vi "Periodic Tasks.vi"(8 "error in":errorcluster) -> (0 "error out":errorcluster)   [LabVIEW 2018]
doc: "This VI runs in parallel to other tasks. It can contain as many user-defined periodic loops as you need. These can carry out PID or other sorts of timed response."
uses:
  <vilib>/Rock Robotics/WPI/Joystick/WPI_JoystickDevRef.ctl
  <vilib>/Rock Robotics/WPI/Joystick/WPI_JoystickDeviceEnum.ctl
  <vilib>/Rock Robotics/WPI/RobotDrive/WPI_RobotDriveDevRef.ctl
  <vilib>/Rock Robotics/WPI/MotorControl/WPI_MotorControlDeviceRef.ctl
  <vilib>/Rock Robotics/WPI/MotorControl/WPI_MotorControlType.ctl
  <vilib>/Rock Robotics/SystemInterfaces/DIO/FPGA_DIOPWMChannel.ctl
  <vilib>/Rock Robotics/WPI/PWM/WPI_PWMDeadband.ctl
  <vilib>/Rock Robotics/SystemInterfaces/DIO/FPGA_DIOChannel.ctl
  <vilib>/Rock Robotics/WPI/Solenoid/WPI_SolenoidDevRef.ctl
  <vilib>/Rock Robotics/WPI/Solenoid/WPI_SolenoidChannel.ctl
  <vilib>/Rock Robotics/WPI/DriverStation/WPI_DriverStationRobotMode2.ctl
  Vision States.ctl
  <vilib>/Rock Robotics/WPI/Utilities/WPI_GetSetVariantRefNum.vi
  Robot Global Data.vi
  <vilib>/Rock Robotics/Network Tables/NT Write Number.vi
  <vilib>/Rock Robotics/Network Tables/NT Read Number.vi
panel:
  in  "RetainerSolenoidDevRef":T1={"DevStatus"={"status"=FALSE, "code"=0, "source"=""}, "Pneumatics Control Module"=0, "Forward Solenoid Channel"=enum."Invalid", "Reverse Solenoid Channel"=enum."Invalid"}
  in  "KickerSolenoidDevRef":T1={"DevStatus"={"status"=FALSE, "code"=0, "source"=""}, "Pneumatics Control Module"=0, "Forward Solenoid Channel"=enum."Invalid", "Reverse Solenoid Channel"=enum."Invalid"}
  in  "Drive Motors":T3={"DevStatus"={"status"=FALSE, "code"=0, "source"=""}, "Motors[]"=[], "Square Inputs"=FALSE, "Max Output"=1.0}
  in  "AuxJoystickDevRef":T9={"Device"=enum."USB 1"}
  in  "DriveJoystickDevRef":T9
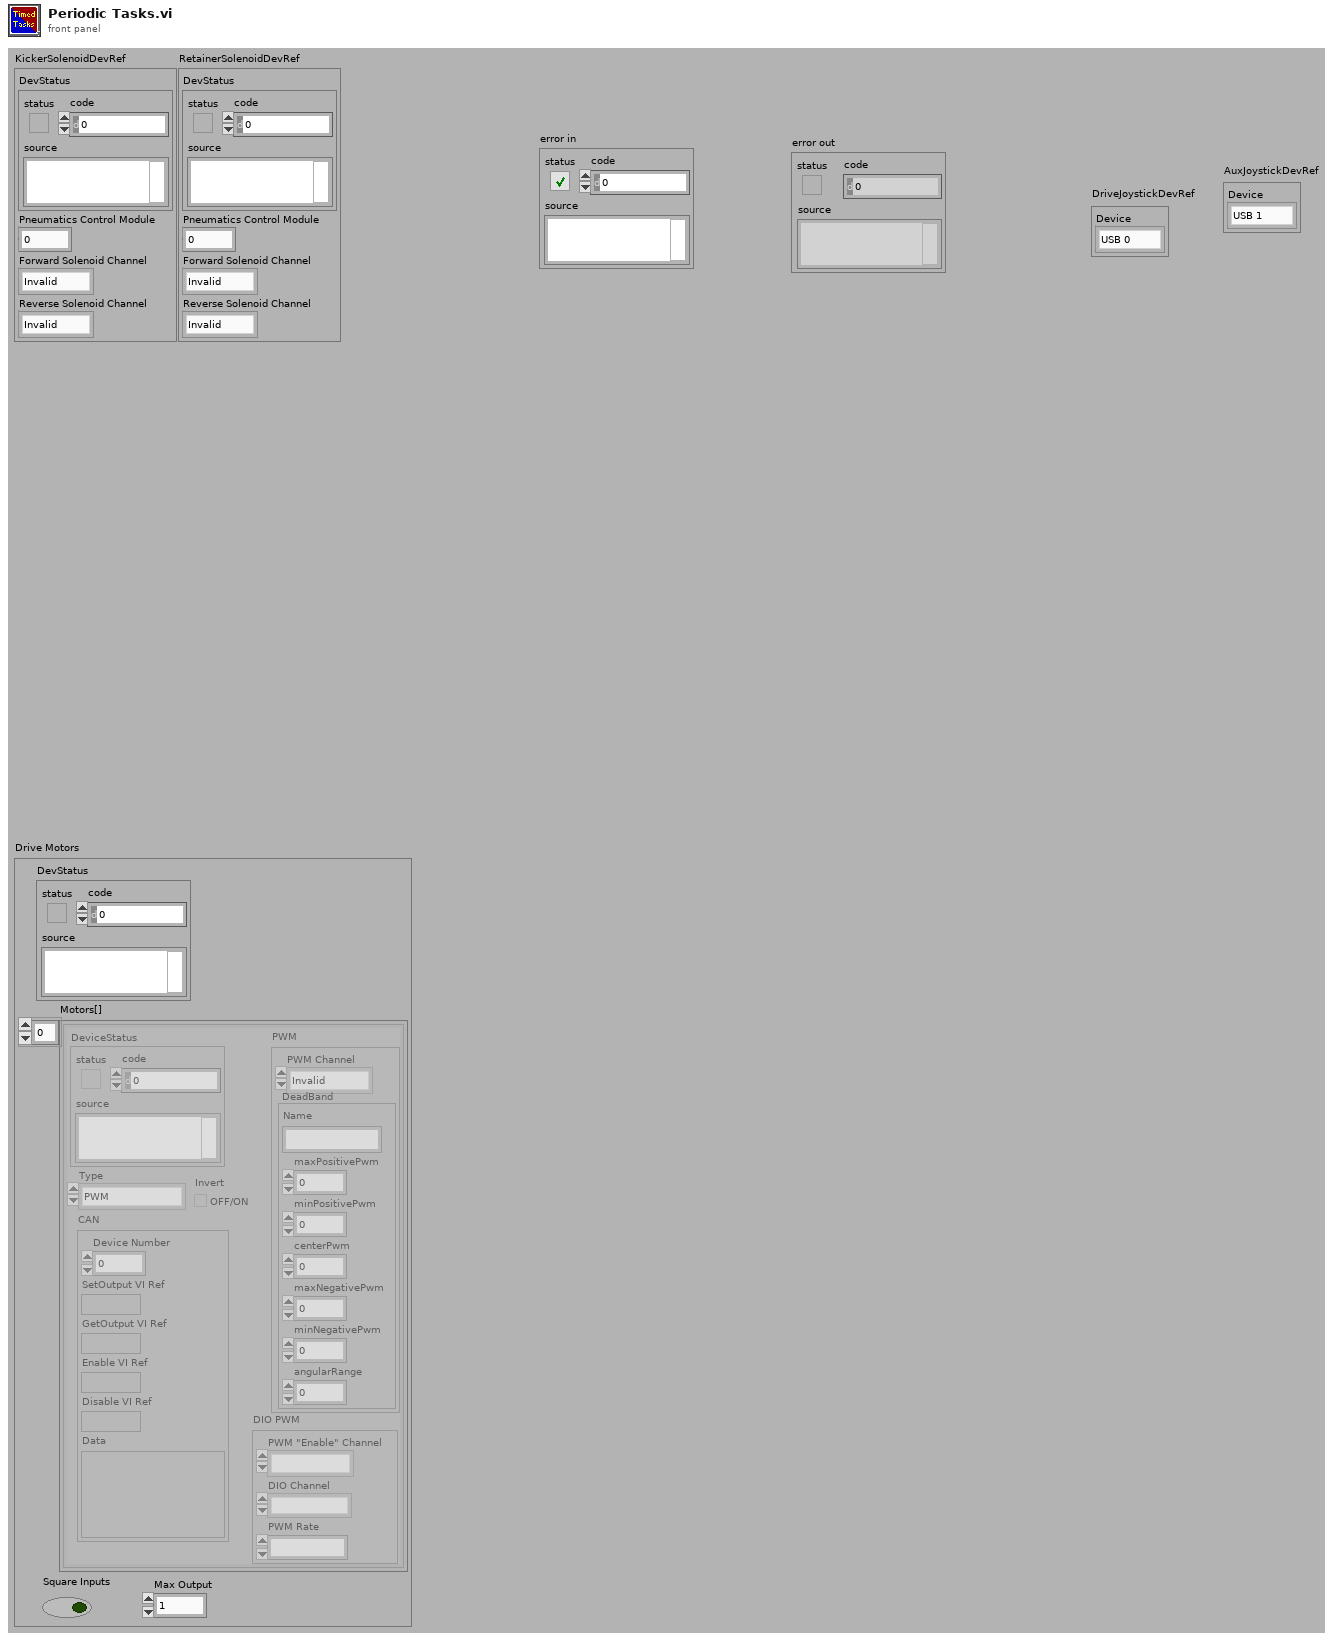
[diagram p1: front panel]
types:
  T1 = typedef "WPI_SolenoidDevRef.ctl" = cluster{"DevStatus":errorcluster, "Pneumatics Control Module":u8, "Forward Solenoid Channel":T2, "Reverse Solenoid Channel":T2}
  T2 = typedef "WPI_SolenoidChannel.ctl" = enum8{"Solenoid 0", "Solenoid 1", "Solenoid 2", "Solenoid 3", "Solenoid 4", "Solenoid 5", "Solenoid 6", "Solenoid 7", "Invalid"}
  T3 = typedef "WPI_RobotDriveDevRef.ctl" = cluster{"DevStatus":errorcluster, "Motors[]":T4[], "Square Inputs":bool, "Max Output":dbl}
  T4 = typedef "WPI_MotorControlDeviceRef.ctl" = cluster{"DeviceStatus":errorcluster, "Type":T5, "PWM":cluster{"PWM Channel":T6, "DeadBand":T7}, "CAN":cluster{"Device Number":u8, "SetOutput VI Ref":variant, "GetOutput VI Ref":variant, "Enable VI Ref":variant, "Disable VI Ref":variant, "Data":variant}, "Invert":bool, "DIO PWM":cluster{"PWM \"Enable\" Channel":T6, "DIOChannel":T8, "PWM Rate":dbl}}
  T5 = typedef "WPI_MotorControlType.ctl" = enum16{"PWM", "CAN", "DIO PWM"}
  T6 = typedef "FPGA_DIOPWMChannel.ctl" = enum8{"PWM 0", "PWM 1", "PWM 2", "PWM 3", "PWM 4", "PWM 5", "PWM 6", "PWM 7", "PWM 8", "PWM 9", "PWM MXP 0", "PWM MXP 1", "PWM MXP 2", "PWM MXP 3", "PWM MXP 4", "PWM MXP 5", "PWM MXP 6", "PWM MXP 7", "PWM MXP 8", "PWM MXP 9", "Invalid"}
  T7 = typedef "WPI_PWMDeadband.ctl" = cluster{"Name":string, "maxPositivePwm":i32, "minPositivePwm":i32, "centerPwm":i32, "maxNegativePwm":i32, "minNegativePwm":i32, "angularRange":u16}
  T8 = typedef "FPGA_DIOChannel.ctl" = enum8{"DIO 0", "DIO 1", "DIO 2", "DIO 3", "DIO 4", "DIO 5", "DIO 6", "DIO 7", "DIO 8", "DIO 9", "DIO MXP 0", "DIO MXP 1", "DIO MXP 2", "DIO MXP 3", "DIO MXP 4", "DIO MXP 5", "DIO MXP 6", "DIO MXP 7", "DIO MXP 8", "DIO MXP 9", "DIO MXP 10", "DIO MXP 11", "DIO MXP 12", "DIO MXP 13", "DIO MXP 14", "DIO MXP 15", "SPI Port CS1", "SPI Port CS2", "SPI Port CS3", "SPI Port MISO", "SPI Port MOSI", "Invalid"}
  T9 = typedef "WPI_JoystickDevRef.ctl" = cluster{"Device":T10}
  T10 = typedef "WPI_JoystickDeviceEnum.ctl" = enum16{"USB 0", "USB 1", "USB 2", "USB 3", "USB 4", "USB 5"}
  T11 = cluster{"offsetAngle H":dbl, "offsetAngle V":dbl, "area":dbl, "skew":dbl, "shortest side (pxls)":dbl, "longest side (pxls)":dbl}
  T12 = typedef "Vision States.ctl" = enum16{"Ready", "Forward Until Target at Edge", "Vision Track"}
  T13 = cluster{"A Button":i32, "B Button":i32, "X Button":i32, "Y Button":i32, "LB Button":i32, "RB Button":i32, "BACK Button":i32, "START Button":i32, "LJ Click Button":i32, "RJ Click Button":i32}
  T14 = cluster{"Left X":i32, "Left Y":i32, "Right X":i32, "Right Y":i32}
  T15 = typedef "WPI_DriverStationRobotMode2.ctl" = enum16{"Autonomous Disabled", "Autonomous Enabled", "Teleop Disabled", "Teleop Enabled", "Disconnected", "Finish", "Test Disabled", "Test Enabled", "Emergency Stopped"}
  T16 = cluster{"KickerSolenoidDevRef":T1, "RetainerSolenoidDevRef":T1}
  T17 = cluster{"DriveJoystickDevRef":T9, "AuxJoystickDevRef":T9, "Drive Axes":dbl[], "Drive Buttons":bool[], "Drive POVs":i16[], "Aux Axes":dbl[], "Aux Buttons":bool[], "Aux POVs":i16[], "Robot Mode":T15, "Drive Motors":T3, "Drive Joystick Indexes":cluster{"Left X":i32, "Left Y":i32, "Right X":i32, "Right Y":i32}, "Drive Button Indexes":cluster{"A Button":i32, "B Button":i32, "X Button":i32, "Y Button":i32, "LB Button":i32, "RB Button":i32, "BACK Button":i32, "START Button":i32, "LJ Click Button":i32, "RJ Click Button":i32}, "Joystick VS Vision Latch":bool, "Vision States":T12, "limelight":cluster{"offsetAngle H":dbl, "offsetAngle V":dbl, "area":dbl, "skew":dbl, "shortest side (pxls)":dbl, "longest side (pxls)":dbl}, "Vision Track Mode Override":bool}
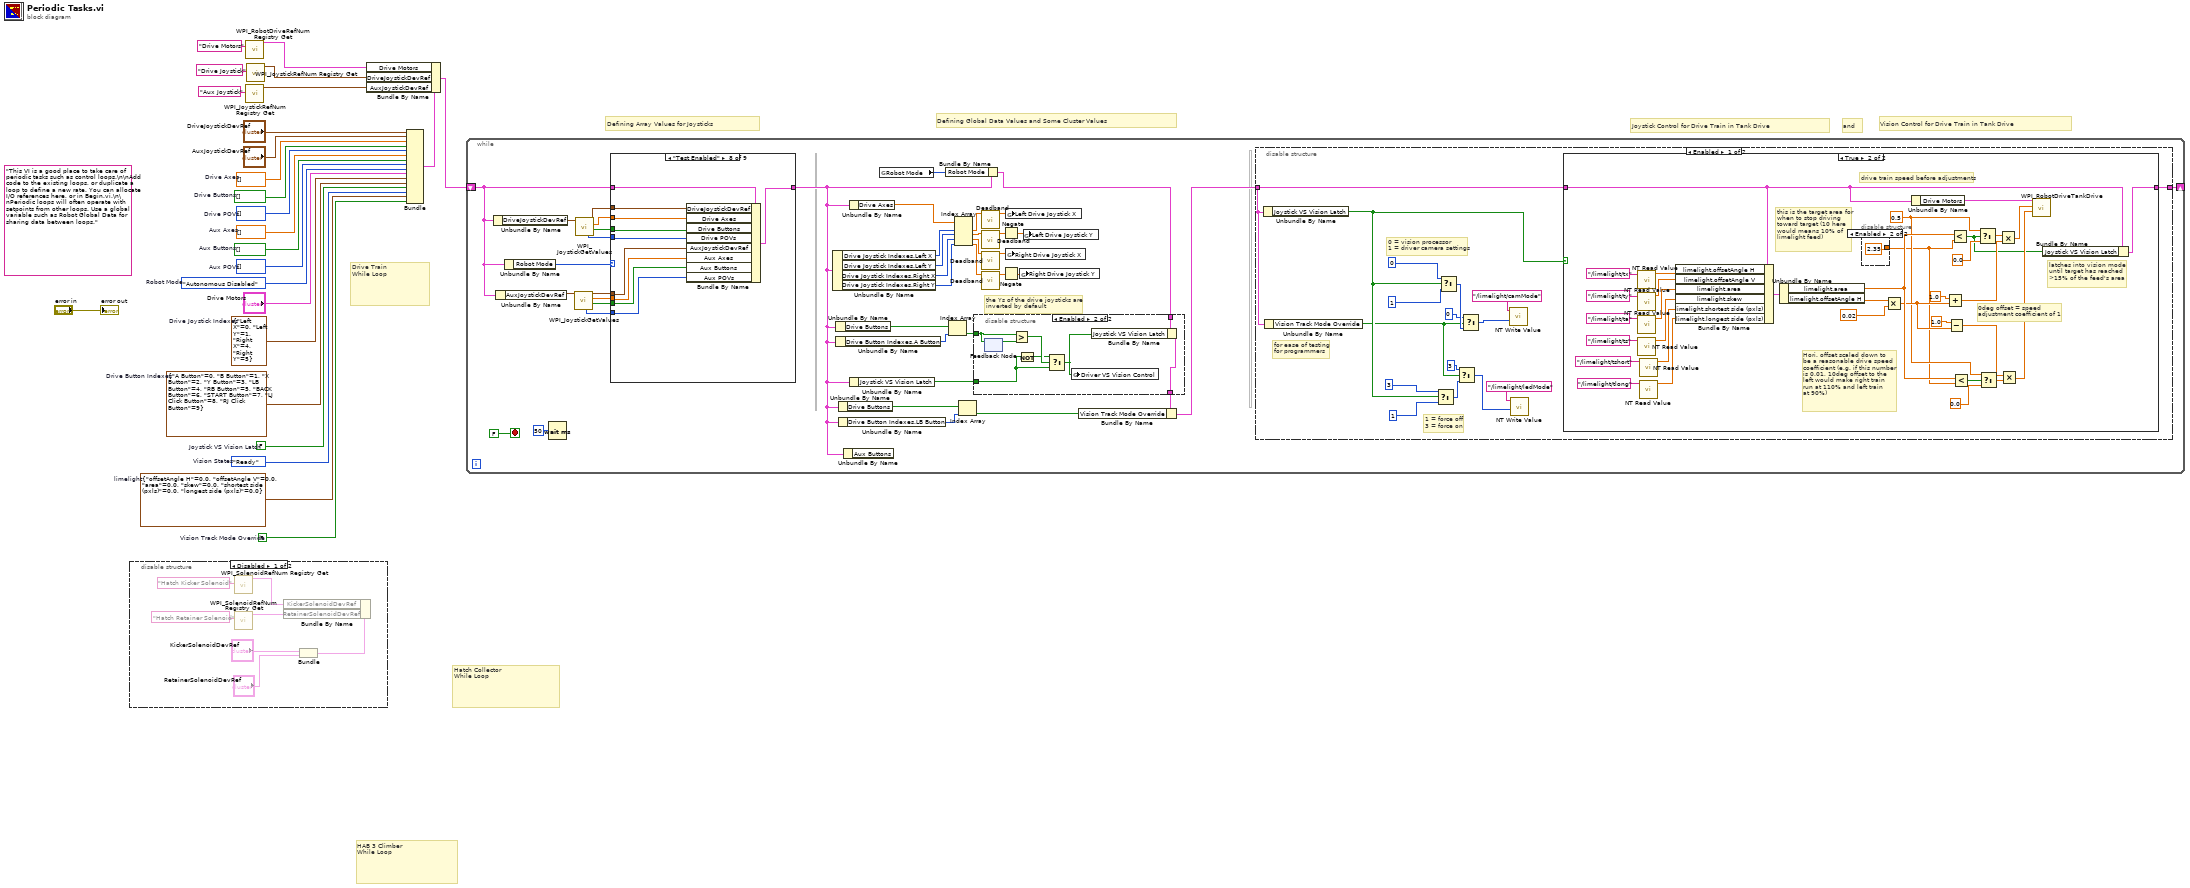
[diagram p0: block diagram]
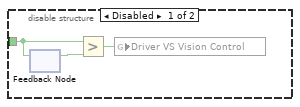
[diagram p3: hidden frame]
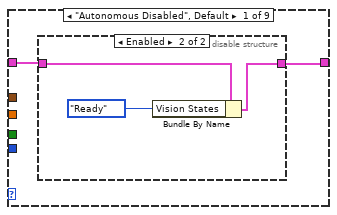
[diagram p4: hidden frame]
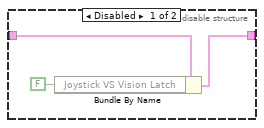
[diagram p5: hidden frame]
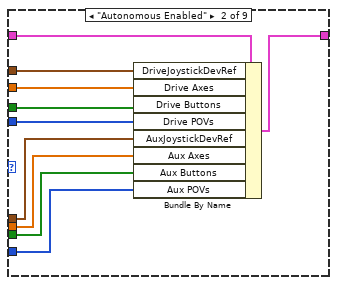
[diagram p6: hidden frame]
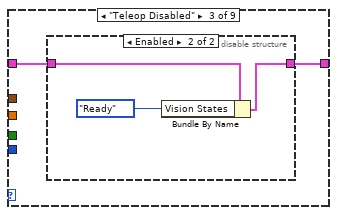
[diagram p7: hidden frame]
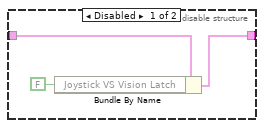
[diagram p8: hidden frame]
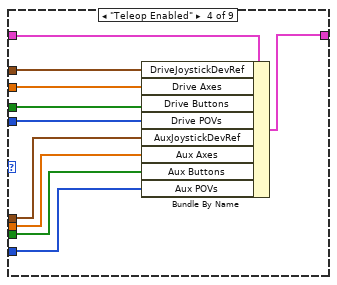
[diagram p9: hidden frame]
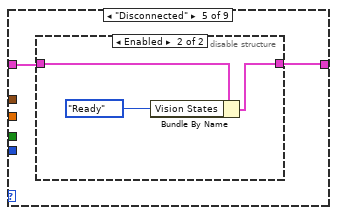
[diagram p10: hidden frame]
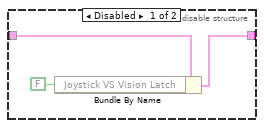
[diagram p11: hidden frame]
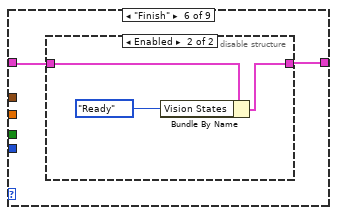
[diagram p12: hidden frame]
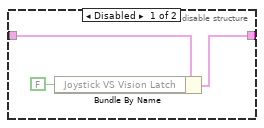
[diagram p13: hidden frame]
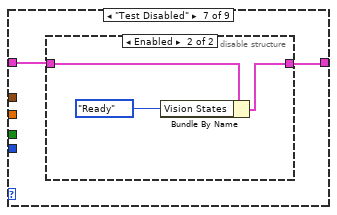
[diagram p14: hidden frame]
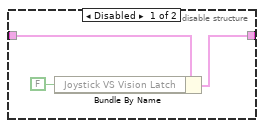
[diagram p15: hidden frame]
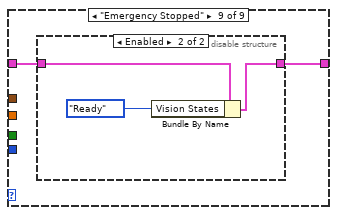
[diagram p16: hidden frame]
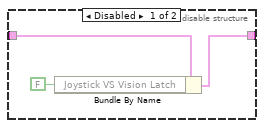
[diagram p17: hidden frame]
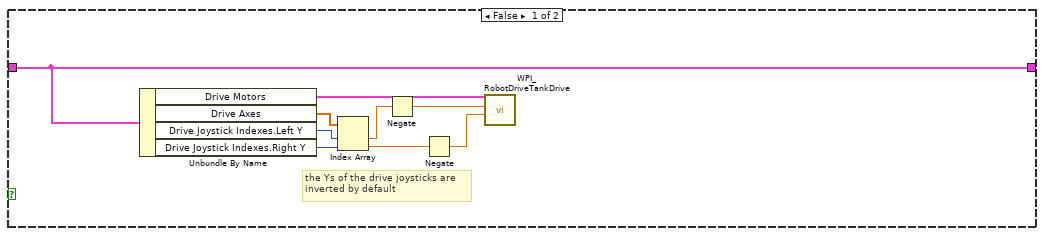
[diagram p18: hidden frame]
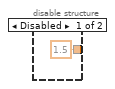
[diagram p19: hidden frame]
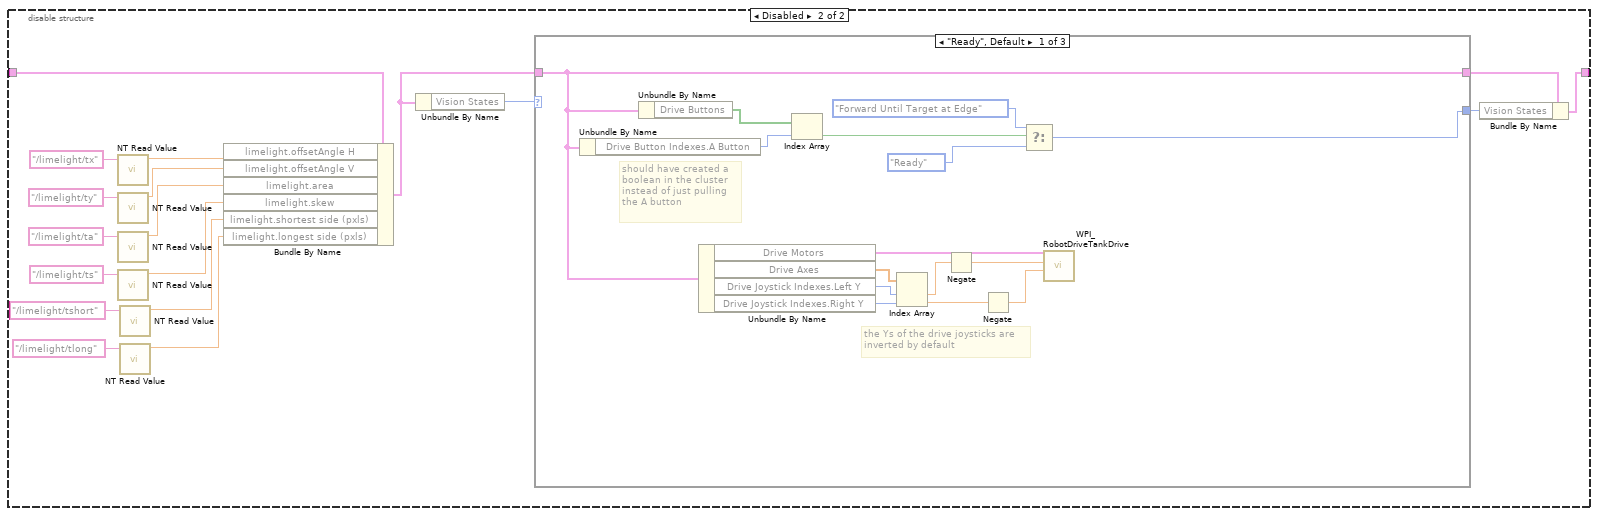
[diagram p20: hidden frame]
diagram:
  w1 = FALSE  # Vision Track Mode Override
  w2 = T11 {"offsetAngle H"=0.0, "offsetAngle V"=0.0, "area"=0.0, "skew"=0.0, "shortest side (pxls)"=0.0, "longest side (pxls)"=0.0}  # limelight
  w3 = Vision_States."Ready"  # Vision States
  w4 = FALSE  # Joystick VS Vision Latch
  w5 = T13 {"A Button"=0, "B Button"=1, "X Button"=2, "Y Button"=3, "LB Button"=4, "RB Button"=5, "BACK Button"=6, "START Button"=7, "LJ Click Button"=8, "RJ Click Button"=9}  # Drive Button Indexes
  w7 = T14 {"Left X"=0, "Left Y"=1, "Right X"=4, "Right Y"=5}  # Drive Joystick Indexes
  w12 = i16[] []  # Aux POVs
  w13 = bool[] []  # Aux Buttons
  w14 = dbl[] []  # Aux Axes
  w11 = WPI_DriverStationRobotMode2."Autonomous Disabled"  # Robot Mode
  w15 = i16[] []  # Drive POVs
  w16 = bool[] []  # Drive Buttons
  w17 = dbl[] []  # Drive Axes
  (unwired) "This VI is a good place to take care of periodic tasks such as control loops.\n\nAdd code to the existing loops, or duplicate a loop to define a new rate. You can allocate I/O references here, or in Begin.vi.\n\nPeriodic loops will often operate with setpoints from other loops. Use a global variable such as Robot Global Data for sharing data between loops."
  # "HAB 3 Climber\nWhile Loop"
  # "Hatch Collector\nWhile Loop"
  # "Drive Train\nWhile Loop"
  # "and"
  # "Vision Control for Drive Train in Tank Drive"
  # "Joystick Control for Drive Train in Tank Drive"
  # "Defining Array Values for Joysticks"
  # "Defining Global Data Values and Some Cluster Values"
  n1 = disable-structure shown="Disabled" {
    frame Disabled {
      n2 = call <vilib>:"WPI_SolenoidRefNum Registry Get.vi"("refnum name"="Hatch Kicker Solenoid") -> ("SolenoidDevRef"=w27:T1)  [unwired: 9 in, 1 out]
      n3 = call <vilib>:"WPI_SolenoidRefNum Registry Get.vi"("refnum name"="Hatch Retainer Solenoid") -> ("SolenoidDevRef"=w26:T1)  [unwired: 9 in, 1 out]
      n4 = Bundle("KickerSolenoidDevRef"="KickerSolenoidDevRef", "RetainerSolenoidDevRef"="RetainerSolenoidDevRef") -> (w30:T16)  [unwired: 1 in]
      n5 = Bundle By Name(cluster=w30, "KickerSolenoidDevRef"=w27, "RetainerSolenoidDevRef"=w26) -> ()  [unwired: 1 out]
    }
    frame Enabled {
    }
  }
  n6 = call <vilib>:"WPI_RobotDriveRefNum Registry Get.vi"("refnum name"="Drive Motors") -> ("RobotDriveDevRef"=w9:T3)  [unwired: 9 in, 1 out]
  n7 = call <vilib>:"WPI_JoystickRefNum Registry Get.vi"("refnum name"="Aux Joystick") -> ("JoystickDevRef"=w19:T9)  [unwired: 9 in, 1 out]
  n8 = call <vilib>:"WPI_JoystickRefNum Registry Get.vi"("refnum name"="Drive Joystick") -> ("JoystickDevRef"=w20:T9)  [unwired: 9 in, 1 out]
  n9 = Bundle("DriveJoystickDevRef"="DriveJoystickDevRef", "AuxJoystickDevRef"="AuxJoystickDevRef", "Drive Axes"=w17, "Drive Buttons"=w16, "Drive POVs"=w15, "Aux Axes"=w14, "Aux Buttons"=w13, "Aux POVs"=w12, "Robot Mode"=w11, "Drive Motors"="Drive Motors", "Drive Joystick Indexes"=w7, "Drive Button Indexes"=w5, "Joystick VS Vision Latch"=w4, "Vision States"=w3, "limelight"=w2, "Vision Track Mode Override"=w1) -> (w21:T17)  [unwired: 1 in]
  n10 = Bundle By Name(cluster=w21, "Drive Motors"=w9, "DriveJoystickDevRef"=w20, "AuxJoystickDevRef"=w19) -> (w18:T17)
  n11 = while {
    shift-right: [w73] -> _
    shift-left: w18 -> [w60]
    stop <- FALSE stop-if-true
    # "the Ys of the drive joysticks are \ninverted by default"
    n12 = Unbundle By Name(w60) -> ("DriveJoystickDevRef"=w71:T9)
    n13 = Unbundle By Name(w60) -> ("AuxJoystickDevRef"=w70:T9)
    n14 = Unbundle By Name(w60) -> ("Robot Mode"=w69:T15)
    n15 = Wait (ms)(milliseconds to wait=u32 50) -> ()  [unwired: 1 out]
    n16 = call <vilib>:"WPI_JoystickGetValues.vi"("JoystickDevRef"=w70) -> ("Buttons"=w62:bool[], "Axes"=w63:dbl[], "JoystickDevRef"=w64:T9, "POVs"=w61:i16[])  [unwired: 6 in, 1 out]
    n17 = call <vilib>:"WPI_JoystickGetValues.vi"("JoystickDevRef"=w71) -> ("Buttons"=w66:bool[], "Axes"=w68:dbl[], "JoystickDevRef"=w67:T9, "POVs"=w65:i16[])  [unwired: 6 in, 1 out]
    n18 = case shown="\"Test Enabled\"" w69 {
      tunnel: w60 -> [w87 w103 w105 w121 w123 w130 w139 w155 w157]
      tunnel: [w86 w94 w104 w112 w122 w131 w138 w146 w156] -> w38
      tunnel: w68 -> [_ w102 _ w119 _ _ _ w153 _]
      tunnel: w67 -> [_ w101 _ w120 _ _ _ w154 _]
      tunnel: w66 -> [_ w100 _ w118 _ _ _ w152 _]
      tunnel: w65 -> [_ w99 _ w117 _ _ _ w151 _]
      tunnel: w64 -> [_ w98 _ w116 _ _ _ w150 _]
      tunnel: w63 -> [_ w97 _ w115 _ _ _ w149 _]
      tunnel: w62 -> [_ w96 _ w114 _ _ _ w148 _]
      tunnel: w61 -> [_ w95 _ w113 _ _ _ w147 _]
      frame "Autonomous Disabled", Default {
        n19 = disable-structure shown="Enabled" {
          disable-tunnel: w87 -> [w89 w93]
          disable-tunnel: [w88 w92] -> w86
          frame Disabled {
            n20 = Bundle By Name(cluster=w89, "Joystick VS Vision Latch"=FALSE) -> (w88:T17)
          }
          frame Enabled {
            n21 = Bundle By Name(cluster=w93, "Vision States"=Vision_States."Ready") -> (w92:T17)
          }
        }
      }
      frame "Autonomous Enabled" {
        n22 = Bundle By Name(cluster=w103, "DriveJoystickDevRef"=w101, "Drive Axes"=w102, "Drive Buttons"=w100, "Drive POVs"=w99, "AuxJoystickDevRef"=w98, "Aux Axes"=w97, "Aux Buttons"=w96, "Aux POVs"=w95) -> (w94:T17)
      }
      frame "Teleop Disabled" {
        n23 = disable-structure shown="Enabled" {
          disable-tunnel: w105 -> [w107 w111]
          disable-tunnel: [w106 w110] -> w104
          frame Disabled {
            n24 = Bundle By Name(cluster=w107, "Joystick VS Vision Latch"=FALSE) -> (w106:T17)
          }
          frame Enabled {
            n25 = Bundle By Name(cluster=w111, "Vision States"=Vision_States."Ready") -> (w110:T17)
          }
        }
      }
      frame "Teleop Enabled" {
        n26 = Bundle By Name(cluster=w121, "DriveJoystickDevRef"=w120, "Drive Axes"=w119, "Drive Buttons"=w118, "Drive POVs"=w117, "AuxJoystickDevRef"=w116, "Aux Axes"=w115, "Aux Buttons"=w114, "Aux POVs"=w113) -> (w112:T17)
      }
      frame "Disconnected" {
        n27 = disable-structure shown="Enabled" {
          disable-tunnel: w123 -> [w125 w129]
          disable-tunnel: [w124 w128] -> w122
          frame Disabled {
            n28 = Bundle By Name(cluster=w125, "Joystick VS Vision Latch"=FALSE) -> (w124:T17)
          }
          frame Enabled {
            n29 = Bundle By Name(cluster=w129, "Vision States"=Vision_States."Ready") -> (w128:T17)
          }
        }
      }
      frame "Finish" {
        n30 = disable-structure shown="Enabled" {
          disable-tunnel: w130 -> [w133 w137]
          disable-tunnel: [w132 w136] -> w131
          frame Disabled {
            n31 = Bundle By Name(cluster=w133, "Joystick VS Vision Latch"=FALSE) -> (w132:T17)
          }
          frame Enabled {
            n32 = Bundle By Name(cluster=w137, "Vision States"=Vision_States."Ready") -> (w136:T17)
          }
        }
      }
      frame "Test Disabled" {
        n33 = disable-structure shown="Enabled" {
          disable-tunnel: w139 -> [w141 w145]
          disable-tunnel: [w140 w144] -> w138
          frame Disabled {
            n34 = Bundle By Name(cluster=w141, "Joystick VS Vision Latch"=FALSE) -> (w140:T17)
          }
          frame Enabled {
            n35 = Bundle By Name(cluster=w145, "Vision States"=Vision_States."Ready") -> (w144:T17)
          }
        }
      }
      frame "Test Enabled" {
        n36 = Bundle By Name(cluster=w155, "DriveJoystickDevRef"=w154, "Drive Axes"=w153, "Drive Buttons"=w152, "Drive POVs"=w151, "AuxJoystickDevRef"=w150, "Aux Axes"=w149, "Aux Buttons"=w148, "Aux POVs"=w147) -> (w146:T17)
      }
      frame "Emergency Stopped" {
        n37 = disable-structure shown="Enabled" {
          disable-tunnel: w157 -> [w159 w163]
          disable-tunnel: [w158 w162] -> w156
          frame Disabled {
            n38 = Bundle By Name(cluster=w159, "Joystick VS Vision Latch"=FALSE) -> (w158:T17)
          }
          frame Enabled {
            n39 = Bundle By Name(cluster=w163, "Vision States"=Vision_States."Ready") -> (w162:T17)
          }
        }
      }
    }
    n40 = Unbundle By Name(w38) -> ("Drive Joystick Indexes.Left X"=w41:i32, "Drive Joystick Indexes.Left Y"=w42:i32, "Drive Joystick Indexes.Right X"=w43:i32, "Drive Joystick Indexes.Right Y"=w44:i32)
    n41 = Unbundle By Name(w38) -> ("Drive Buttons"=w39:bool[])
    n42 = Unbundle By Name(w38) -> ("Drive Button Indexes.A Button"=w56:i32)
    n43 = Unbundle By Name(w38) -> ("Drive Buttons"=w37:bool[])
    n44 = Unbundle By Name(w38) -> ("Drive Button Indexes.LB Button"=w36:i32)
    n45 = Unbundle By Name(w38) -> ()  [unwired: 1 out]
    n46 = Unbundle By Name(w38) -> ("Joystick VS Vision Latch"=w58:bool)
    n47 = Unbundle By Name(w38) -> ("Drive Axes"=w40:dbl[])
    n48 = global read "Robot Global Data.vi" "Robot Mode"() -> (w45:T15)
    n49 = Bundle By Name(cluster=w38, "Robot Mode"=w45) -> (w59:T17)
    n50 = Index Array(array=w39, index=w56) -> (element=w57:bool)
    n51 = Index Array(array=w40, index #1=w41, index #2=w42, index #3=w43, index #4=w44) -> (element #1=w49:dbl, element #2=w50:dbl, element #3=w51:dbl, element #4=w52:dbl)
    n52 = Index Array(array=w37, index=w36) -> (element=w34:bool)
    n53 = disable-structure shown="Enabled" {
      disable-tunnel: w57 -> [w77 w84]
      disable-tunnel: w58 -> [_ w82]
      disable-tunnel: w59 -> [_ w80]
      disable-tunnel: [_ w78] -> w35
      frame Disabled {
        n54 = feedback #1() -> (w76:bool)  [unwired: 1 in]
        n55 = feedback-in #1(w77) -> ()
        n56 = Greater?(x=w77, y=w76) -> (0:w75:bool)
        n57 = global write "Robot Global Data.vi" "Driver VS Vision Control"(w75) -> ()
      }
      frame Enabled {
        n58 = feedback #2() -> (w85:bool)  [unwired: 1 in]
        n59 = feedback-in #2(w84) -> ()
        n60 = Greater?(x=w84, y=w85) -> (0:w83:bool)
        n61 = Not(x=w82) -> (.not. x?=w81:bool)
        n62 = Select(t=w81, s=w83, f=w82) -> (s? t:f=w79:bool)
        n63 = global write "Robot Global Data.vi" "Driver VS Vision Control"(w79) -> ()
        n64 = Bundle By Name(cluster=w80, "Joystick VS Vision Latch"=w79) -> (w78:T17)
      }
    }
    n65 = call "Deadband.vi"("Input"=w49) -> ("Output"=w47:dbl)  [unwired: 10 in]
    n66 = call "Deadband.vi"("Input"=w50) -> ("Output"=w48:dbl)  [unwired: 10 in]
    n67 = call "Deadband.vi"("Input"=w51) -> ("Output"=w46:dbl)  [unwired: 10 in]
    n68 = call "Deadband.vi"("Input"=w52) -> ("Output"=w53:dbl)  [unwired: 10 in]
    n69 = Negate(x=w48) -> (-x=w54:dbl)
    n70 = Negate(x=w53) -> (-x=w55:dbl)
    n71 = global write "Robot Global Data.vi" "Left Drive Joystick X"(w47) -> ()
    n72 = global write "Robot Global Data.vi" "Right Drive Joystick X"(w46) -> ()
    n73 = global write "Robot Global Data.vi" "Right Drive Joystick Y"(w55) -> ()
    n74 = global write "Robot Global Data.vi" "Left Drive Joystick Y"(w54) -> ()
    n75 = Bundle By Name(cluster=w35, "Vision Track Mode Override"=w34) -> (w33:T17)
    n76 = disable-structure shown="Enabled" {
      disable-tunnel: [w179 w240] -> w73
      disable-tunnel: w33 -> [w171 w226]
      frame Enabled {
        # "for ease of testing\nfor programmers"
        # "1 = force off\n3 = force on"
        # "0 = vision processor\n1 = driver camera settings"
        n77 = Unbundle By Name(w171) -> ("Joystick VS Vision Latch"=w175:bool)
        n78 = Unbundle By Name(w171) -> ("Vision Track Mode Override"=w167:bool)
        n79 = Select(t=3, s=w175, f=1) -> (s? t:f=w166:i32)
        n80 = Select(t=0, s=w175, f=1) -> (s? t:f=w170:i32)
        n81 = Select(t=3, s=w167, f=w166) -> (s? t:f=w165:i32)
        n82 = Select(t=0, s=w167, f=w170) -> (s? t:f=w168:i32)
        n83 = call-poly <vilib>:"NT Write Value.vi"("Numeric"=w168, "Name"="/limelight/camMode") -> ()  [unwired: 9 in, 1 out]
        n84 = call-poly <vilib>:"NT Write Value.vi"("Numeric"=w165, "Name"="/limelight/ledMode") -> ()  [unwired: 9 in, 1 out]
        n85 = case shown="True" w175 {
          tunnel: w171 -> [w180 w222]
          tunnel: [w180 w221] -> w179
          frame False {
            # "the Ys of the drive joysticks are \ninverted by default"
            n86 = Unbundle By Name(w180) -> ("Drive Motors"=w188:T3, "Drive Axes"=w187:dbl[], "Drive Joystick Indexes.Left Y"=w186:i32, "Drive Joystick Indexes.Right Y"=w185:i32)
            n87 = Index Array(array=w187, index #1=w186, index #2=w185) -> (element #1=w184:dbl, element #2=w183:dbl)
            n88 = Negate(x=w184) -> (-x=w181:dbl)
            n89 = Negate(x=w183) -> (-x=w182:dbl)
            n90 = call <vilib>:"WPI_RobotDriveTankDrive.vi"("Right axis value"=w182, "Left axis value"=w181, "RobotDriveDevRef"=w188) -> ()  [unwired: 6 in, 3 out]
          }
          frame True {
            w196 = 0.5 ("t")
            # "latches into vision mode \nuntil target has reached \n>15% of the feed's area"
            # "drive train speed before adjustments"
            # "this is the target area for\nwhen to stop driving \ntoward target (10 here \nwould means 10% of \nlimelight feed)"
            # "Hori. offset scaled down to\nbe a reasonable drive speed\ncoefficient (e.g. if this number\nis 0.01, 10deg offset to the \nleft would make right train \nrun at 110% and left train \nat 90%)"
            # "0deg offset = speed \nadjustment coefficient of 1"
            n91 = call-poly <vilib>:"NT Read Value.vi"("Name"="/limelight/tx") -> ("Numeric"=w216:dbl)  [unwired: 9 in, 1 out]
            n92 = call-poly <vilib>:"NT Read Value.vi"("Name"="/limelight/ty") -> ("Numeric"=w215:dbl)  [unwired: 9 in, 1 out]
            n93 = call-poly <vilib>:"NT Read Value.vi"("Name"="/limelight/ta") -> ("Numeric"=w214:dbl)  [unwired: 9 in, 1 out]
            n94 = call-poly <vilib>:"NT Read Value.vi"("Name"="/limelight/ts") -> ("Numeric"=w213:dbl)  [unwired: 9 in, 1 out]
            n95 = call-poly <vilib>:"NT Read Value.vi"("Name"="/limelight/tshort") -> ("Numeric"=w190:dbl)  [unwired: 9 in, 1 out]
            n96 = call-poly <vilib>:"NT Read Value.vi"("Name"="/limelight/tlong") -> ("Numeric"=w189:dbl)  [unwired: 9 in, 1 out]
            n97 = Bundle By Name(cluster=w222, "limelight.offsetAngle H"=w216, "limelight.offsetAngle V"=w215, "limelight.area"=w214, "limelight.skew"=w213, "limelight.shortest side (pxls)"=w190, "limelight.longest side (pxls)"=w189) -> (w212:T17)
            n98 = Unbundle By Name(w212) -> ("limelight.area"=w201:dbl, "limelight.offsetAngle H"=w209:dbl)
            n99 = disable-structure shown="Enabled" {
              disable-tunnel: [1.5 2.35] -> w195
              frame Disabled {
              }
              frame Enabled {
              }
            }
            n100 = Multiply(x=w209, y=0.02) -> (x*y=w198:dbl)
            n101 = Unbundle By Name(w222) -> ("Drive Motors"=w194:T3)
            n102 = Add(x=1.0, y=w198) -> (x+y=w204:dbl)
            n103 = Subtract(x=1.0, y=w198) -> (x-y=w197:dbl)
            n104 = Less?(x=w201, y=w195) -> (x < y?=w193:bool)
            n105 = Less?(x=w201, y=w195) -> (x < y?=w205:bool)
            n106 = Select(t=w196, s=w193, f=0.0) -> (s? t:f=w210:dbl)
            n107 = Select(t=w196, s=w205, f=0.0) -> (s? t:f=w202:dbl)
            n108 = Multiply(x=w210, y=w204) -> (x*y=w207:dbl)
            n109 = Multiply(x=w197, y=w202) -> (x*y=w200:dbl)
            n110 = call <vilib>:"WPI_RobotDriveTankDrive.vi"("Right axis value"=w200, "Left axis value"=w207, "RobotDriveDevRef"=w194) -> ()  [unwired: 6 in, 3 out]
            n111 = Bundle By Name(cluster=w222, "Joystick VS Vision Latch"=w193) -> (w221:T17)
          }
        }
      }
      frame Disabled {
        n112 = call-poly <vilib>:"NT Read Value.vi"("Name"="/limelight/tx") -> ("Numeric"=w234:dbl)  [unwired: 9 in, 1 out]
        n113 = call-poly <vilib>:"NT Read Value.vi"("Name"="/limelight/ty") -> ("Numeric"=w233:dbl)  [unwired: 9 in, 1 out]
        n114 = call-poly <vilib>:"NT Read Value.vi"("Name"="/limelight/ta") -> ("Numeric"=w232:dbl)  [unwired: 9 in, 1 out]
        n115 = call-poly <vilib>:"NT Read Value.vi"("Name"="/limelight/ts") -> ("Numeric"=w231:dbl)  [unwired: 9 in, 1 out]
        n116 = call-poly <vilib>:"NT Read Value.vi"("Name"="/limelight/tshort") -> ("Numeric"=w228:dbl)  [unwired: 9 in, 1 out]
        n117 = call-poly <vilib>:"NT Read Value.vi"("Name"="/limelight/tlong") -> ("Numeric"=w227:dbl)  [unwired: 9 in, 1 out]
        n118 = Bundle By Name(cluster=w226, "limelight.offsetAngle H"=w234, "limelight.offsetAngle V"=w233, "limelight.area"=w232, "limelight.skew"=w231, "limelight.shortest side (pxls)"=w228, "limelight.longest side (pxls)"=w227) -> (w225:T17)
        n119 = Unbundle By Name(w225) -> ("Vision States"=w242:T12)
        n120 = case shown="\"Ready\", Default" w242 {
          tunnel: [w243 w258 w276] -> w241
          tunnel: w225 -> [w243 w258 w276]
          tunnel: [w252 w259 w272] -> w239
          frame "Ready", Default {
            # "should have created a \nboolean in the cluster \ninstead of just pulling\nthe A button"
            # "the Ys of the drive joysticks are \ninverted by default"
            n121 = Unbundle By Name(w243) -> ("Drive Button Indexes.A Button"=w257:i32)
            n122 = Unbundle By Name(w243) -> ("Drive Buttons"=w256:bool[])
            n123 = Unbundle By Name(w243) -> ("Drive Motors"=w251:T3, "Drive Axes"=w250:dbl[], "Drive Joystick Indexes.Left Y"=w249:i32, "Drive Joystick Indexes.Right Y"=w248:i32)
            n124 = Index Array(array=w256, index=w257) -> (element=w255:bool)
            n125 = Index Array(array=w250, index #1=w249, index #2=w248) -> (element #1=w247:dbl, element #2=w246:dbl)
            n126 = Negate(x=w247) -> (-x=w244:dbl)
            n127 = Negate(x=w246) -> (-x=w245:dbl)
            n128 = Select(t=Vision_States."Forward Until Target at Edge" ("Vision States"), s=w255, f=Vision_States."Ready" ("Vision States")) -> (s? t:f=w252:T12)
            n129 = call <vilib>:"WPI_RobotDriveTankDrive.vi"("Right axis value"=w245, "Left axis value"=w244, "RobotDriveDevRef"=w251) -> ()  [unwired: 6 in, 3 out]
          }
          frame "Forward Until Target at Edge" {
            n130 = Unbundle By Name(w258) -> ("limelight.offsetAngle H"=w263:dbl)
            n131 = Less?(x=w263, y=-26) -> (x < y?=w261:bool)
            n132 = Greater?(x=w263, y=14) -> (0:w262:bool)
            n133 = Or(x=w262, y=w261) -> (x .or. y?=w260:bool)
            n134 = case shown="False" w260 {
              tunnel: [Vision_States."Forward Until Target at Edge" ("Vision States") Vision_States."Vision Track" ("Vision States")] -> w259
              tunnel: w258 -> [w269 _]
              frame False {
                w267 = 0.35
                n135 = Unbundle By Name(w269) -> ("Drive Motors"=w268:T3)
                n136 = call <vilib>:"WPI_RobotDriveTankDrive.vi"("Right axis value"=w267, "Left axis value"=w267, "RobotDriveDevRef"=w268) -> ()  [unwired: 6 in, 3 out]
              }
              frame True {
              }
            }
          }
          frame "Vision Track" {
            w279 = 0.5 ("t")
            w278 = 1.5
            # "this is the target area for\nwhen to stop driving \ntoward target (10 here \nwould means 10% of \nlimelight feed)"
            # "Hori. offset scaled down to\nbe a reasonable drive speed\ncoefficient (e.g. if this number\nis 0.01, 10deg offset to the \nleft would make right train \nrun at 110% and left train \nat 90%)"
            # "0deg offset = speed \nadjustment coefficient of 1"
            n137 = Unbundle By Name(w276) -> ("limelight.area"=w284:dbl, "limelight.offsetAngle H"=w292:dbl)
            n138 = Multiply(x=w292, y=0.03) -> (x*y=w281:dbl)
            n139 = Unbundle By Name(w276) -> ("Drive Motors"=w277:T3)
            n140 = Add(x=1.0, y=w281) -> (x+y=w287:dbl)
            n141 = Subtract(x=1.0, y=w281) -> (x-y=w280:dbl)
            n142 = Less?(x=w284, y=w278) -> (x < y?=w275:bool)
            n143 = Less?(x=w284, y=w278) -> (x < y?=w288:bool)
            n144 = Select(t=w279, s=w275, f=0.0) -> (s? t:f=w293:dbl)
            n145 = Select(t=w279, s=w288, f=0.0) -> (s? t:f=w285:dbl)
            n146 = Multiply(x=w293, y=w287) -> (x*y=w290:dbl)
            n147 = Multiply(x=w280, y=w285) -> (x*y=w283:dbl)
            n148 = Not(x=w275) -> (.not. x?=w271:bool)
            n149 = call <vilib>:"WPI_RobotDriveTankDrive.vi"("Right axis value"=w283, "Left axis value"=w290, "RobotDriveDevRef"=w277) -> ()  [unwired: 6 in, 3 out]
            n150 = Select(t=Vision_States."Ready" ("Vision States"), s=w271, f=Vision_States."Vision Track" ("Vision States")) -> (s? t:f=w272:T12)
          }
        }
        n151 = Bundle By Name(cluster=w241, "Vision States"=w239) -> (w240:T17)
      }
    }
  }
  "error out" <- "error in"
